vi "Write X11.vi"(5 "Username":string, 6 "Password":string, 7 "Address":string, 8 "Error In":errorcluster) -> (0 "Error Out":errorcluster)   [LabVIEW 2018, in "Tests.lvlib" / "Channel.lvlib"]
uses:
  Channel.lvlib
  src/Toolkit/API/Channel/Channel.lvclass/Channel.ctl
  src/Toolkit/API/Session/Session.lvclass/Session.ctl
  src/Toolkit/API/SSH/SSH.lvclass/SSH.ctl
  src/Toolkit/API/Session/Utility/Read Shared Library.vi
  src/Toolkit/API/SSH/Utility/Read Shared Library.vi
  src/Toolkit/Support/Check Status.vi
  <vilib>/addons/_JKI Toolkits/Caraya/classes/Test/Test.lvclass
  <vilib>/addons/_JKI Toolkits/Caraya/classes/Assert/Assert.lvclass
  src/Toolkit/API/Channel/Channel.lvclass
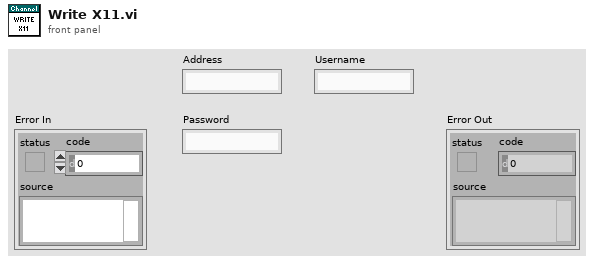
[diagram p1: front panel]
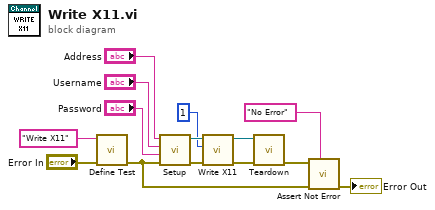
[diagram p0: block diagram]
diagram:
  n1 = call <vilib>:"Define Test.vi"("error in (no error)"="Error In", "Label (VI Title)"="Write X11") -> ("error out"=w11:errorcluster)  [unwired: 9 in]
  n2 = call "Setup.vi"("Error In"=w11, "Password"="Password", "Username"="Username", "Address"="Address") -> ("Error Out"=w4:errorcluster, "Channel"=w5:refnum<class "Channel.lvclass">)  [unwired: 6 in]
  n3 = call "Write X11.vi"("Error In"=w4, "Screen"=1, "Channel In"=w5) -> ("Error Out"=w3:errorcluster, "Channel Out"=w2:refnum<class "Channel.lvclass">)  [unwired: 7 in]
  n4 = call "Teardown.vi"("Error In"=w3, "Channel"=w2) -> ("Error Out"=w7:errorcluster)  [unwired: 9 in]
  n5 = call <vilib>:"Assert Not Error.vi"("Label"="No Error", "error in (no error)"=w11, "Not Error?"=w7) -> ("error out"=→"Error Out":errorcluster)  [unwired: 8 in]
